vi "RM.forceDeleteReservation.vi"(7 "Resource Type":T1, 8 "error in":errorcluster, 10 "name in bitfile":string, 11 "reservation DB in":variant) -> (0 "error out":errorcluster, 2 "found?":bool, 3 "reservation DB out":variant)   [LabVIEW 2016, in "FPGA Resource Manager.lvlib"]
uses:
  FPGA Resource Manager.lvlib
  RM.resourceType.ctl
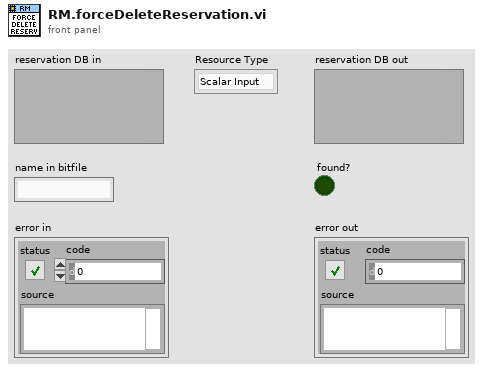
[diagram p1: front panel]
types:
  T1 = typedef "FPGA Resource Manager.lvlib/RM.resourceType.ctl" = enum16{"Scalar Input", "Scalar Output", "Waveform Input", "Waveform Output"}
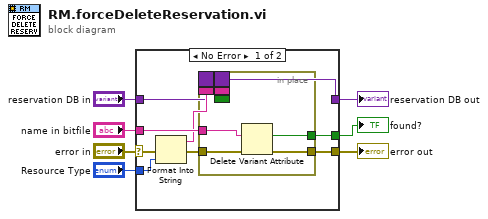
[diagram p0: block diagram]
diagram:
  n1 = case shown="No Error" "error in" {
    selector: "error in" -> [w14 w23]
    tunnel: "reservation DB in" -> [w9 w24]
    tunnel: [w8 w24] -> w1
    tunnel: "name in bitfile" -> [w16 _]
    tunnel: "Resource Type" -> [w15 _]
    tunnel: [w13 w23] -> w3
    tunnel: [w12 _] -> w2
    frame No Error {
      n2 = Format Into String(error in=w14, w15) -> (resulting string=w10:string, error out=w11:errorcluster)  [unwired: 2 in]
      n3 = in-place {
        in-place-border: w16 -> [w19]
        in-place-border: [w21] -> w13
        in-place-border: [w20] -> w12
        border: w9 -> [_]
        border: w10 -> [_]
        border: [_] -> w8
        border: _ -> [_]
        border: _ -> [_]
        in-place-border: w11 -> [w17]
        n4 = Delete Variant Attribute(4:w17, 6:w19, 7:w18) -> (0:w21:errorcluster, 2:w20:bool, 3:w22:variant)
      }
    }
    frame Error {
    }
  }
  "reservation DB out" <- w1
  "error out" <- w3
  "found?" <- w2
